vi "运维调试.vi"() -> ()   [LabVIEW 2016]
uses:
  <vilib>/Utility/sysdir.llb/System Directory Type.ctl
  <vilib>/Utility/miscctls.llb/LVPointTypeDef.ctl
  PLC/PLC.lvlib
  <vilib>/Utility/config.llb/NI_LVConfig.lvlib
panel:
  in  "运维调试菜单":T1(xcontrol)
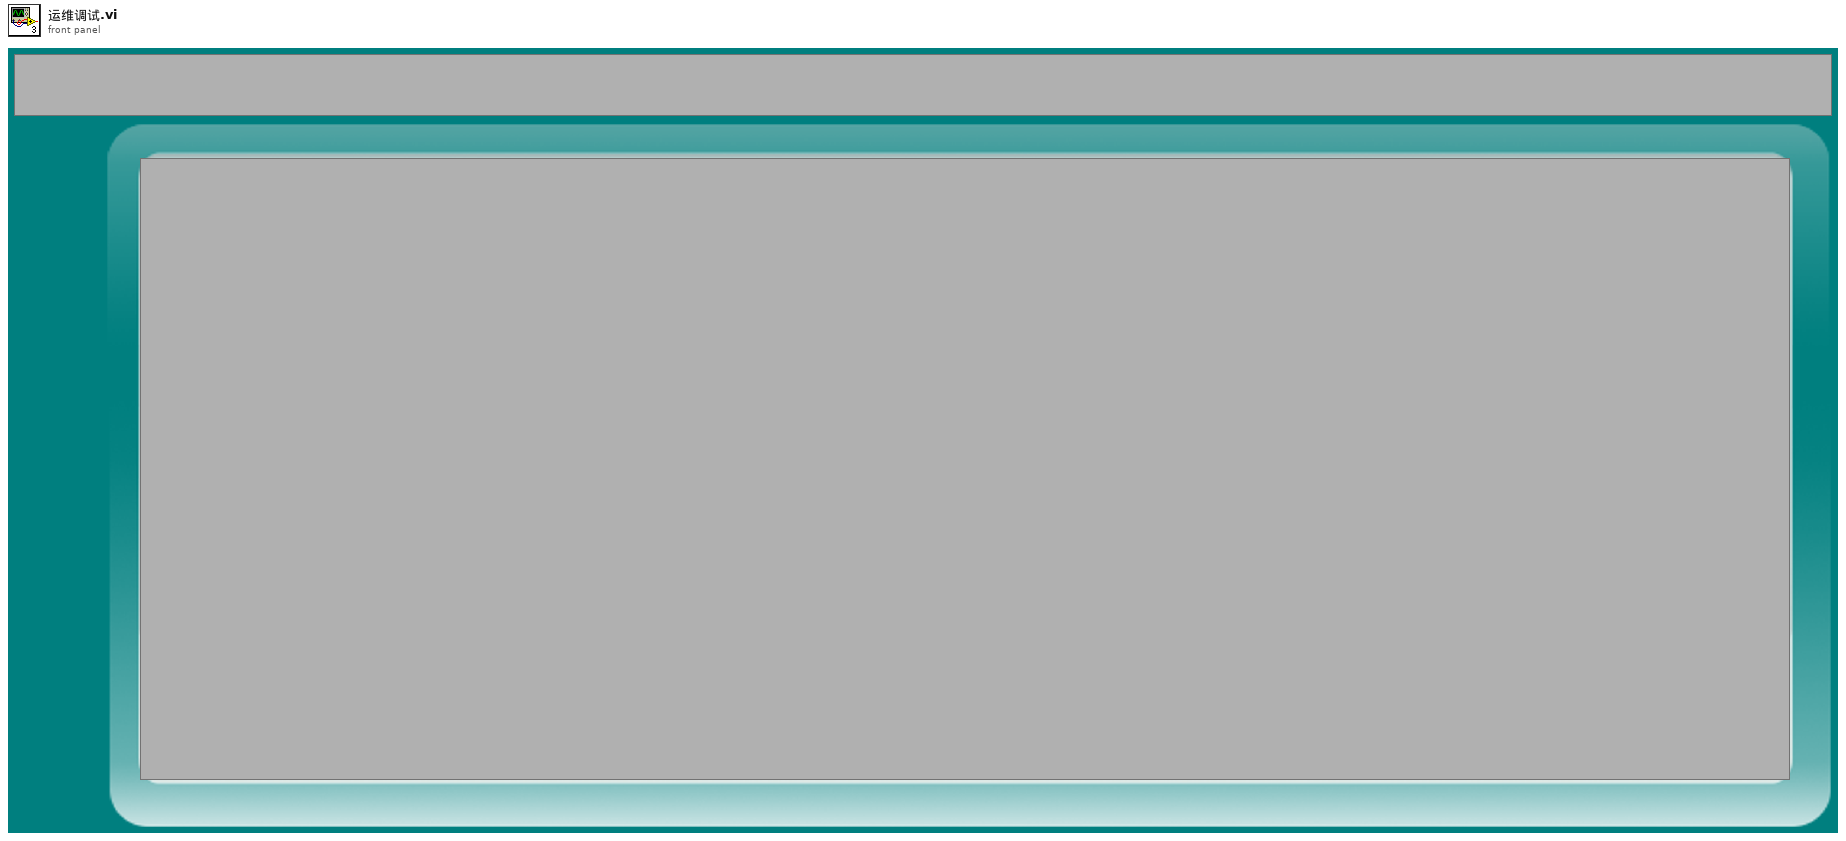
[diagram p1: front panel]
types:
  T1 = enum16{"采配水", "氨氮", "总磷", "总氮", "多参数", "CODMn", "CODcr", "流量计", "质控单元", "超标留样", "其他"}
  T2 = typedef "System Directory Type.ctl" = i32
  T3 = typedef "NI_LVConfig.lvlib/Config Data RefNum.ctl" = refnum<k1>
  T4 = typedef "LVPointTypeDef.ctl" = cluster{"Horizontal":i16, "Vertical":i16}
  T5 = enum16{"Enabled", "Disabled", "Disabled and Grayed Out"}
  T6 = enum32{"Bad", "Idle", "Run top level", "Running"}
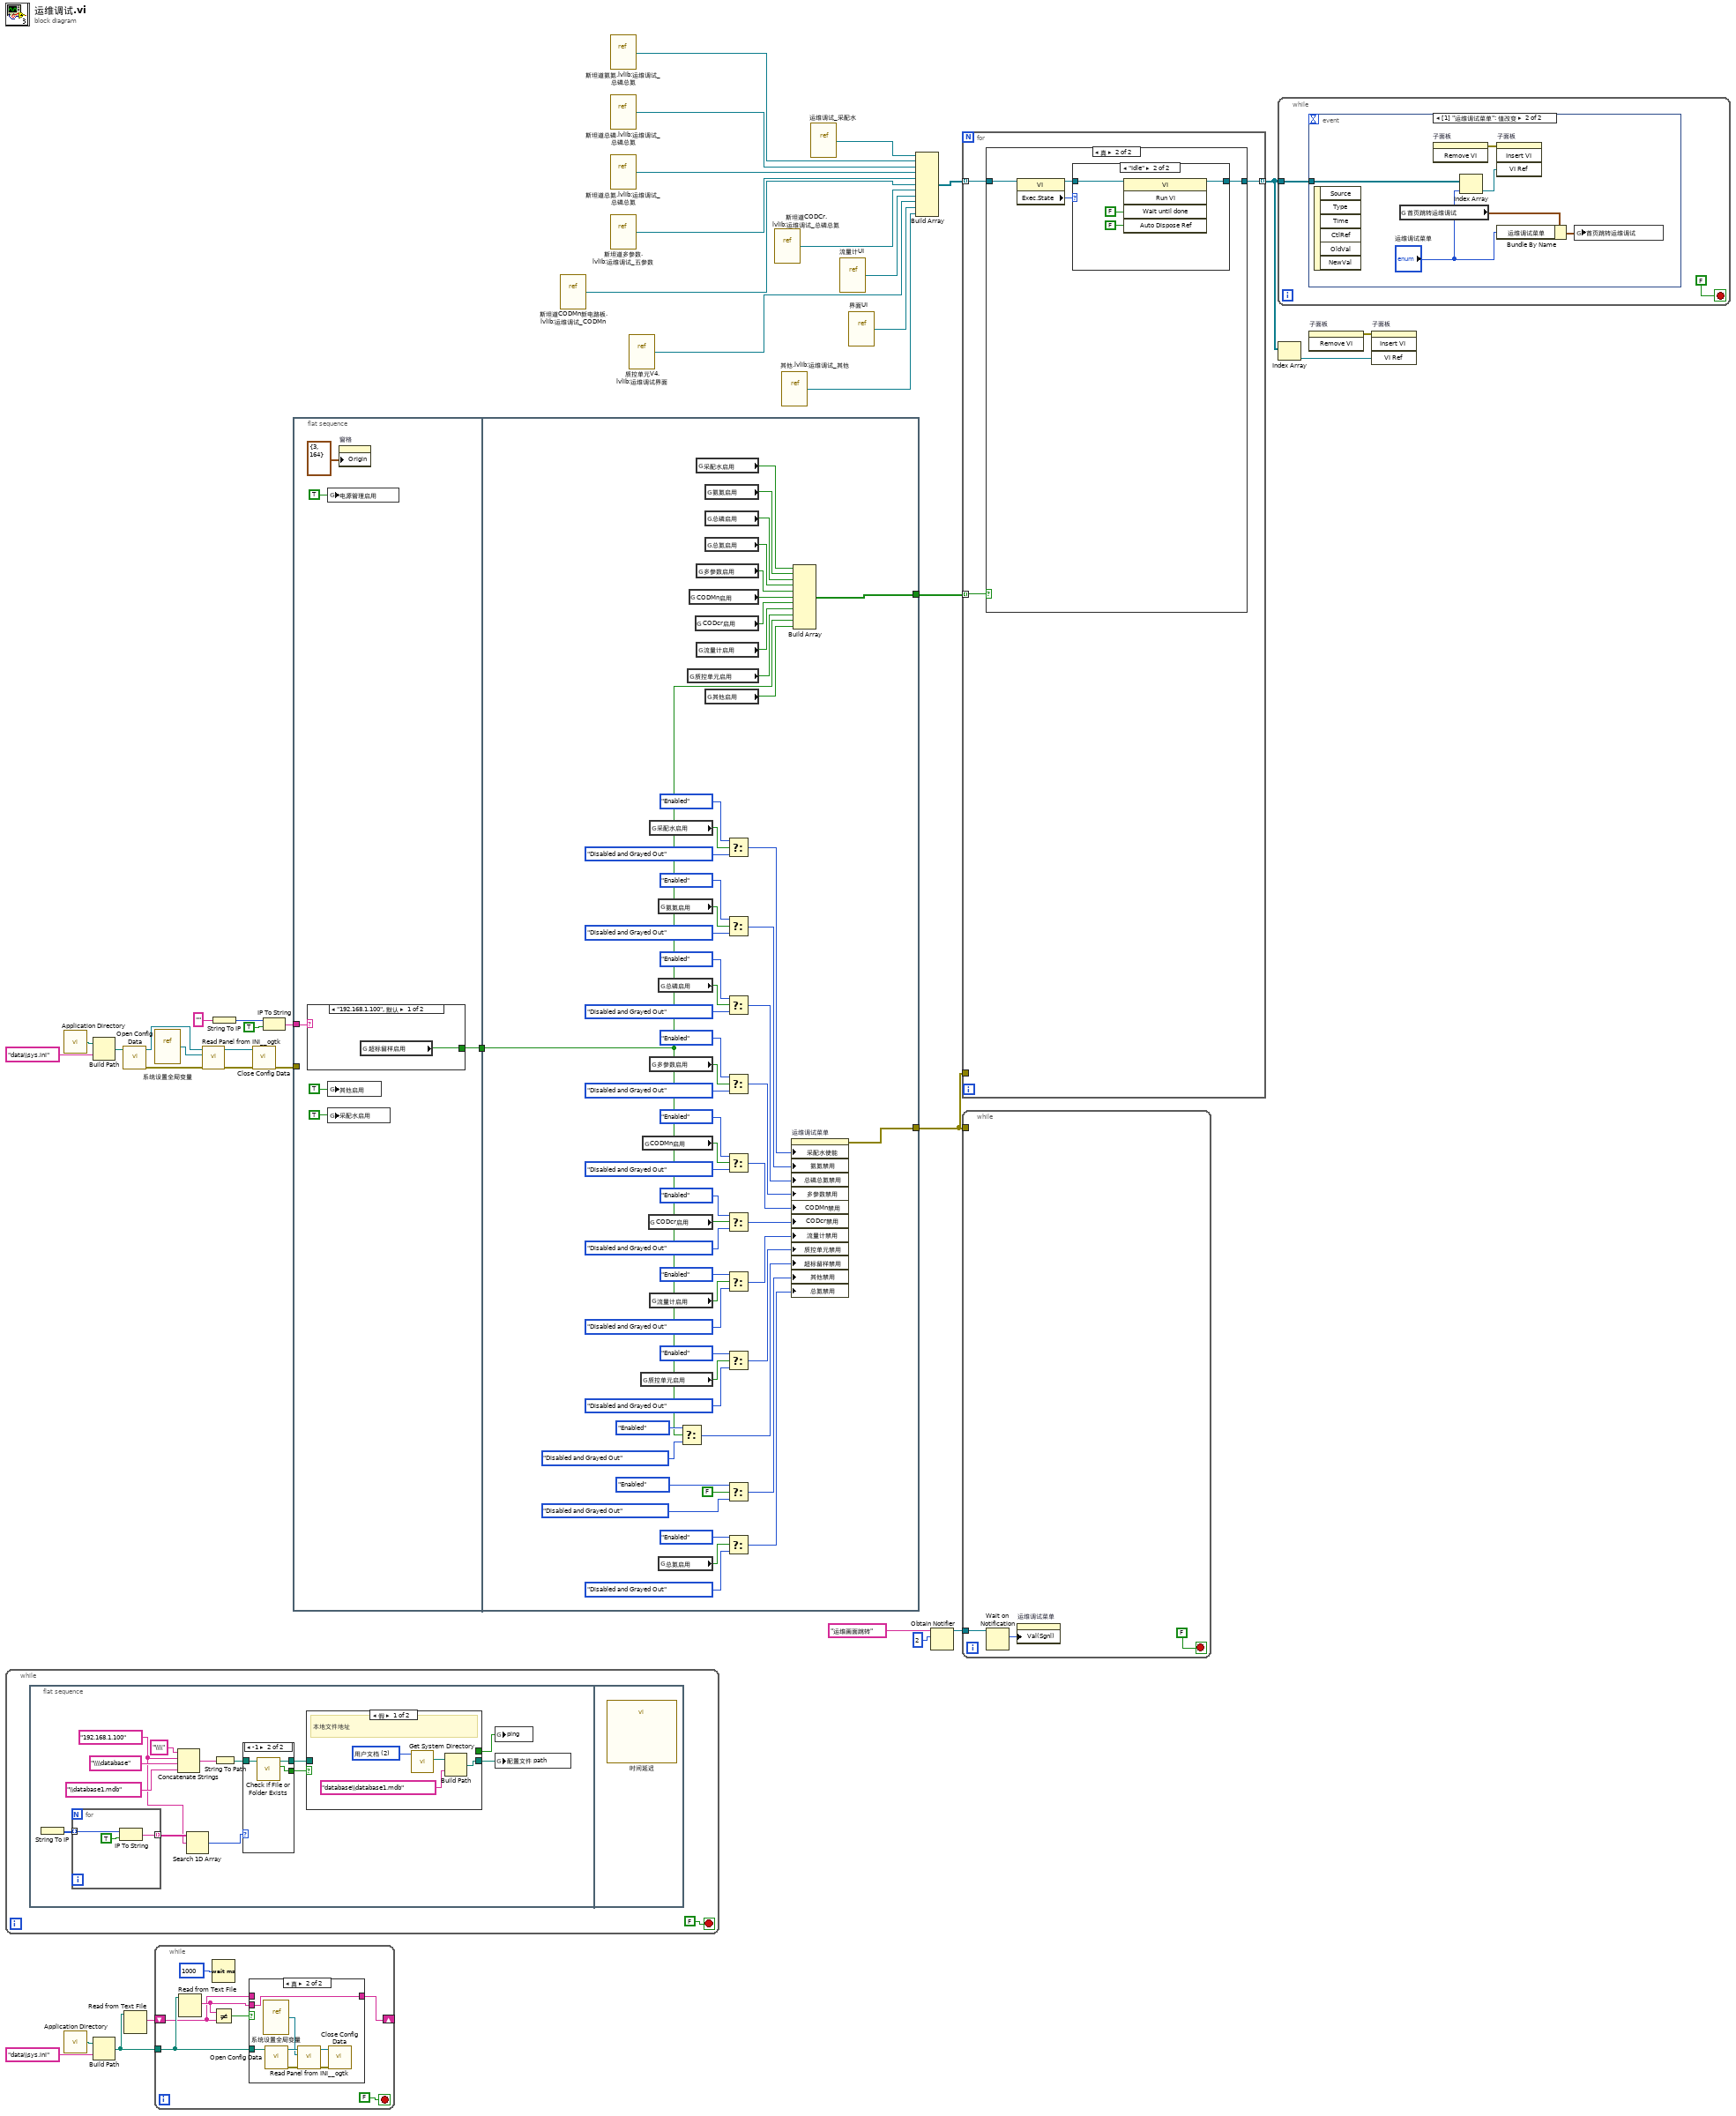
[diagram p0: block diagram]
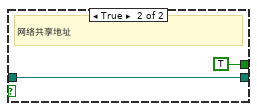
[diagram p2: hidden frame]
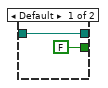
[diagram p3: hidden frame]
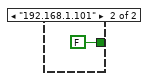
[diagram p5: hidden frame]
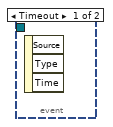
[diagram p8: hidden frame]
diagram:
  n1 = while {
    stop <- FALSE stop-if-true
    n2 = flat-sequence {
      frame #0 {
        w45 = "192.168.1.100" ("名称")
        n3 = String To IP() -> (0:w47:u32[])  [unwired: 1 in]
        n4 = for {
          tunnel: w47 -> [w61] mode=indexing
          tunnel: [w59] -> w46 mode=indexing
          n5 = IP To String(1:TRUE ("句点符号？(F)"), 2:w61) -> (0:w59:string)
        }
        n6 = Concatenate Strings("\\\\" ("字符串"), w45, "\\\\database" ("字符串"), "\\database1.mdb" ("名称或相对路径")) -> (w51:string)
        n7 = Search 1D Array(1D array=w46, element=w45) -> (index of element=w44:i32)  [unwired: 1 in]
        n8 = String To Path(string=w51) -> (path=w48:path)
        n9 = case shown="-1" w44 {
          tunnel: w48 -> [w62 w66]
          tunnel: [w62 w65] -> w43
          tunnel: [FALSE w64] -> w42
          frame Default {
          }
          frame -1 {
            n10 = call <vilib>:"Check if File or Folder Exists.vi"("path"=w66) -> ("file or folder exists?"=w64:bool, "dup path"=w65:path)  [unwired: 8 in, 1 out]
          }
        }
        n11 = case shown="假" w42 {
          tunnel: w43 -> [_ w58]
          tunnel: [w55 w58] -> w41
          tunnel: [_ TRUE] -> w40
          frame False {
            w53 = T2 2 items=["用户目录"=0, "用户桌面"=1, "用户文档"=2, "用户应用程序数据"=3, "用户设置"=4, "用户临时目录"=5, "公共文档"=6, "公共应用程序数据"=7, "公共设置"=8, "公共缓存"=13, "系统核心库"=9, "系统安装库"=10, "应用程序文件"=11, "启动盘根目录"=12] ("system directory type")
            # "本地文件地址"
            n12 = call <vilib>:"Get System Directory.vi"("system directory type"=w53) -> ("system directory"=w54:path)  [unwired: 10 in]
            n13 = Build Path(base path=w54, name or relative path="database\\database1.mdb" ("名称或相对路径")) -> (appended path=w55:path)
          }
          frame True {
            # "网络共享地址"
          }
        }
        n14 = global write "ping全局.vi" "ping"(w40) -> ()
        n15 = global write "ping全局.vi" "配置文件 path"(w41) -> ()
      }
      frame #1 {
        n16 = call "时间延迟"() -> ()  [unwired: 11 in, 1 out]
      }
    }
  }
  n17 = call <vilib>:"Application Directory.vi"() -> ("Application Directory"=w1:path)
  n18 = call <vilib>:"Application Directory.vi"() -> ("Application Directory"=w7:path)
  n19 = Build Path(base path=w1, name or relative path="data\\sys.ini" ("名称或相对路径")) -> (appended path=w3:path)
  n20 = Build Path(base path=w7, name or relative path="data\\sys.ini" ("名称或相对路径")) -> (appended path=w4:path)
  n21 = call <vilib>:"Open Config Data.vi"("configuration file path"=w3) -> ("error out"=w31:errorcluster, "refnum"=w30:T3)  [unwired: 8 in, 1 out]
  n22 = Read from Text File(file (use dialog)=w4) -> (text=w5:string)  [unwired: 3 in, 3 out]
  n23 = vi-ref "系统设置全局变量.vi"() -> (w29:refnum<vi>)
  n24 = while {
    shift-right: [w69] -> _
    shift-left: w5 -> [w68]
    tunnel: w4 -> [w72]
    stop <- FALSE stop-if-true
    n25 = Read from Text File(file (use dialog)=w72) -> (text=w70:string)  [unwired: 3 in, 3 out]
    n26 = Wait (ms)(milliseconds to wait=u32 1000 ("等待时间（毫秒）")) -> ()  [unwired: 1 out]
    n27 = Not Equal?(x=w70, y=w68) -> (x != y?=w73:bool)
    n28 = case shown="真" w73 {
      tunnel: w72 -> [_ w76]
      tunnel: w70 -> [_ w75]
      tunnel: [w74 w75] -> w69
      tunnel: w68 -> [w74 _]
      frame False {
      }
      frame True {
        n29 = vi-ref "系统设置全局变量.vi"() -> (w79:refnum<vi>)
        n30 = call <vilib>:"Open Config Data.vi"("configuration file path"=w76) -> ("error out"=w81:errorcluster, "refnum"=w80:T3)  [unwired: 8 in, 1 out]
        n31 = call <userlib>:"Read Panel from INI__ogtk.vi"("error in (no error)"=w81, "VI ref"=w79, "refnum"=w80) -> ("error out"=w78:errorcluster, "refnum out"=w77:T3)  [unwired: 7 in]
        n32 = call <vilib>:"Close Config Data.vi"("error in (no error)"=w78, "refnum"=w77) -> ()  [unwired: 8 in, 2 out]
      }
    }
  }
  n33 = call <userlib>:"Read Panel from INI__ogtk.vi"("error in (no error)"=w31, "VI ref"=w29, "refnum"=w30) -> ("error out"=w28:errorcluster, "refnum out"=w27:T3)  [unwired: 7 in]
  n34 = String To IP(1:"" ("名称")) -> (0:w17:u32)
  n35 = call <vilib>:"Close Config Data.vi"("error in (no error)"=w28, "refnum"=w27) -> ("error out"=w8:errorcluster)  [unwired: 8 in, 1 out]
  n36 = IP To String(1:TRUE ("句点符号？(F)"), 2:w17) -> (0:w9:string)
  n37 = flat-sequence {
    tunnel: w9 -> [w83]
    tunnel: [w82] -> w14
    tunnel: w8 -> [_]
    tunnel: [w130] -> w10
    tunnel: [w127] -> w26
    tunnel: w14 -> [w90]
    frame #0 {
      n38 = case shown="\"192.168.1.100\", 默认" w83 {
        tunnel: [w88 FALSE] -> w82
        frame "192.168.1.100", Default {
          n39 = global read "系统设置全局变量.vi" "超标留样启用"() -> (w88:bool)
        }
        frame "192.168.1.101" {
        }
      }
      n40 = global write "系统设置全局变量.vi" "电源管理启用"(TRUE ("电源管理启用")) -> ()
      n41 = global write "系统设置全局变量.vi" "其他启用"(TRUE ("其他启用")) -> ()
      n42 = global write "系统设置全局变量.vi" "采配水启用"(TRUE ("采配水启用")) -> ()
      n43 = property on="窗格" class="Pane"("Origin"=T4 {"Horizontal"=3, "Vertical"=164} ("原点")) -> ()  [unwired: 2 in, 2 out]
    }
    frame #1 {
      n44 = global read "系统设置全局变量.vi" "质控单元启用"() -> (w135:bool)
      n45 = global read "系统设置全局变量.vi" "CODMn启用"() -> (w138:bool)
      n46 = global read "系统设置全局变量.vi" "CODcr启用"() -> (w137:bool)
      n47 = global read "系统设置全局变量.vi" "采配水启用"() -> (w144:bool)
      n48 = global read "系统设置全局变量.vi" "多参数启用"() -> (w140:bool)
      n49 = global read "系统设置全局变量.vi" "流量计启用"() -> (w136:bool)
      n50 = global read "系统设置全局变量.vi" "氨氮启用"() -> (w143:bool)
      n51 = global read "系统设置全局变量.vi" "总磷启用"() -> (w92:bool)
      n52 = global read "系统设置全局变量.vi" "总氮启用"() -> (w94:bool)
      n53 = Select(t=T5."Enabled" ("电源管理禁用"), s=w90, f=T5."Disabled and Grayed Out" ("电源管理禁用")) -> (s? t:f=w105:T5)
      n54 = global read "系统设置全局变量.vi" "质控单元启用"() -> (w98:bool)
      n55 = global read "系统设置全局变量.vi" "CODMn启用"() -> (w101:bool)
      n56 = global read "系统设置全局变量.vi" "CODcr启用"() -> (w100:bool)
      n57 = global read "系统设置全局变量.vi" "采配水启用"() -> (w128:bool)
      n58 = global read "系统设置全局变量.vi" "多参数启用"() -> (w102:bool)
      n59 = global read "系统设置全局变量.vi" "流量计启用"() -> (w99:bool)
      n60 = global read "系统设置全局变量.vi" "氨氮启用"() -> (w129:bool)
      n61 = global read "系统设置全局变量.vi" "总磷启用"() -> (w104:bool)
      n62 = global read "系统设置全局变量.vi" "总氮启用"() -> (w103:bool)
      n63 = global read "系统设置全局变量.vi" "其他启用"() -> (w97:bool)
      n64 = Select(t=T5."Enabled" ("电源管理禁用"), s=w144, f=T5."Disabled and Grayed Out" ("电源管理禁用")) -> (s? t:f=w145:T5)
      n65 = Select(t=T5."Enabled" ("电源管理禁用"), s=w143, f=T5."Disabled and Grayed Out" ("电源管理禁用")) -> (s? t:f=w142:T5)
      n66 = Select(t=T5."Enabled" ("电源管理禁用"), s=w92, f=T5."Disabled and Grayed Out" ("电源管理禁用")) -> (s? t:f=w141:T5)
      n67 = Select(t=T5."Enabled" ("电源管理禁用"), s=w140, f=T5."Disabled and Grayed Out" ("电源管理禁用")) -> (s? t:f=w139:T5)
      n68 = Select(t=T5."Enabled" ("电源管理禁用"), s=w138, f=T5."Disabled and Grayed Out" ("电源管理禁用")) -> (s? t:f=w134:T5)
      n69 = Select(t=T5."Enabled" ("电源管理禁用"), s=w137, f=T5."Disabled and Grayed Out" ("电源管理禁用")) -> (s? t:f=w133:T5)
      n70 = Select(t=T5."Enabled" ("电源管理禁用"), s=w136, f=T5."Disabled and Grayed Out" ("电源管理禁用")) -> (s? t:f=w132:T5)
      n71 = Select(t=T5."Enabled" ("电源管理禁用"), s=w135, f=T5."Disabled and Grayed Out" ("电源管理禁用")) -> (s? t:f=w131:T5)
      n72 = Select(t=T5."Enabled" ("电源管理禁用"), s=FALSE, f=T5."Disabled and Grayed Out" ("电源管理禁用")) -> (s? t:f=w108:T5)
      n73 = Select(t=T5."Enabled" ("电源管理禁用"), s=w94, f=T5."Disabled and Grayed Out" ("电源管理禁用")) -> (s? t:f=w93:T5)
      n74 = property on="运维调试菜单" class="运维调试菜单 (严格)"("采配水使能"=w145, "氨氮禁用"=w142, "总磷总氮禁用"=w141, "多参数禁用"=w139, "CODMn禁用"=w134, "CODcr禁用"=w133, "流量计禁用"=w132, "质控单元禁用"=w131, "超标留样禁用"=w105, "其他禁用"=w108, "总氮禁用"=w93) -> (error out=w130:errorcluster)  [unwired: 2 in, 1 out]
      n75 = Build Array(w128, w129, w104, w103, w102, w101, w100, w99, w98, w90, w97) -> (w127:bool[])
    }
  }
  n76 = vi-ref "斯坦道CODMn新电路板.lvlib:运维调试_CODMn.vi"() -> (w23:refnum<vi>)
  n77 = vi-ref "斯坦道氨氮.lvlib:运维调试_总磷总氮.vi"() -> (w33:refnum<vi>)
  n78 = vi-ref "斯坦道总磷.lvlib:运维调试_总磷总氮.vi"() -> (w32:refnum<vi>)
  n79 = vi-ref "斯坦道总氮.lvlib:运维调试_总磷总氮.vi"() -> (w25:refnum<vi>)
  n80 = vi-ref "斯坦道多参数.lvlib:运维调试_五参数.vi"() -> (w24:refnum<vi>)
  n81 = vi-ref "质控单元V4.lvlib:运维调试界面.vi"() -> (w20:refnum<vi>)
  n82 = vi-ref "斯坦道CODCr.lvlib:运维调试_总磷总氮.vi"() -> (w22:refnum<vi>)
  n83 = vi-ref "其他.lvlib:运维调试_其他.vi"() -> (w18:refnum<vi>)
  n84 = vi-ref "运维调试_采配水.vi"() -> (w34:refnum<vi>)
  n85 = vi-ref "流量计UI.vi"() -> (w21:refnum<vi>)
  n86 = vi-ref "界面UI.vi"() -> (w19:refnum<vi>)
  n87 = Build Array(w34, w33, w32, w25, w24, w23, w22, w21, w20, w19, w18) -> (w35:refnum<vi>[])
  n88 = Obtain Notifier(name (unnamed)="运维画面跳转" ("名称（未命名）"), notification data type=2 ("主画面菜单")) -> (notifier out=w11:refnum<notifier>)  [unwired: 2 in, 2 out]
  n89 = for {
    tunnel: w35 -> [w148] mode=indexing
    tunnel: [w147] -> w37 mode=indexing
    tunnel: w26 -> [w146] mode=indexing
    tunnel: w10 -> [_]
    n90 = case shown="真" w146 {
      tunnel: w148 -> [w149 w153]
      tunnel: [w149 w150] -> w147
      frame False {
      }
      frame True {
        n91 = property class="VI"(reference=w153) -> (reference out=w151:refnum<vi>, "Exec.State"=w152:T6)  [unwired: 1 in, 1 out]
        n92 = case shown="\"Idle\"" w152 {
          tunnel: w151 -> [w154 w156]
          tunnel: [w154 w155] -> w150
          frame "Bad", Default {
          }
          frame "Idle" {
            n93 = invoke class="VI" method="Run VI"(reference=w156, "Wait until done"=FALSE ("结束前等待"), "Auto Dispose Ref"=FALSE ("自动销毁引用")) -> (reference out=w155:refnum<vi>)  [unwired: 2 in, 4 out]
          }
        }
      }
    }
  }
  n94 = while {
    tunnel: w11 -> [w161]
    tunnel: w10 -> [_]
    stop <- FALSE stop-if-true
    n95 = Wait on Notification(notifier=w161) -> (notification=w160:i32)  [unwired: 3 in, 3 out]
    n96 = property on="运维调试菜单" class="运维调试菜单 (严格)"("Val(Sgnl)"=w160) -> ()  [unwired: 2 in, 2 out]
  }
  n97 = while {
    tunnel: w37 -> [w162]
    stop <- FALSE stop-if-true
    n98 = event shown="[1] \"运维调试菜单\": 值改变" {
      selector: _ -> [_ _]
      dyn-events: _ -> [_ _]
      timeout: _ -> [_ _]
      tunnel: w162 -> [_ w168]
      event Timeout {
        n99 = event-data() -> ()  [unwired: 1 in, 3 out]
      }
      event "运维调试菜单": Value Change {
        n100 = event-data() -> ()  [unwired: 1 in, 6 out]
        n101 = global read "系统设置全局变量.vi" "首页跳转运维调试"() -> (w166:cluster{"主画面菜单":i32, "运维调试菜单":i32})
        n102 = invoke on="子面板" class="SubPnl" method="Remove VI"() -> (error out=w169:errorcluster)  [unwired: 3 in, 2 out]
        n103 = Index Array(array=w168, index="运维调试菜单") -> (element=w167:refnum<vi>)
        n104 = invoke on="子面板" class="SubPnl" method="Insert VI"(error in=w169, "VI Ref"=w167) -> ()  [unwired: 2 in, 4 out]
        n105 = Bundle By Name(cluster=w166, "运维调试菜单"="运维调试菜单") -> (w165:cluster{"主画面菜单":i32, "运维调试菜单":i32})
        n106 = global write "系统设置全局变量.vi" "首页跳转运维调试"(w165) -> ()
      }
    }
  }
  n107 = Index Array(array=w37) -> (element=w36:refnum<vi>)  [unwired: 1 in]
  n108 = invoke on="子面板" class="SubPnl" method="Remove VI"() -> (error out=w38:errorcluster)  [unwired: 3 in, 2 out]
  n109 = invoke on="子面板" class="SubPnl" method="Insert VI"(error in=w38, "VI Ref"=w36) -> ()  [unwired: 2 in, 4 out]
